vi "Enqueue Element.vi"(7 "timeout in ms (-1)":i32, 8 "error in":errorcluster, 9 "Element Placement":enum16{"To the Front", "To the Back"}(ring), 10 "Q Element":variant, 11 "QueueMessageTransport in":refnum<class "QueueMessageTransport.lvclass">) -> (0 "error out":errorcluster, 3 "QueueMessageTransport out":refnum<class "QueueMessageTransport.lvclass">)   [LabVIEW 2016, in "QueueMessageTransport.lvclass"]
doc: "This public method adds a queue element either <B>to the front</B> of the queue or <B>to the back</B>\n\n**Author: Stas Legedza"
uses:
  QueueMessageTransport.lvclass
  QueueMessageTransport.lvclass/QueueMessageTransport.ctl
panel:
  # "INPUTS"
  # "OUTPUTS"
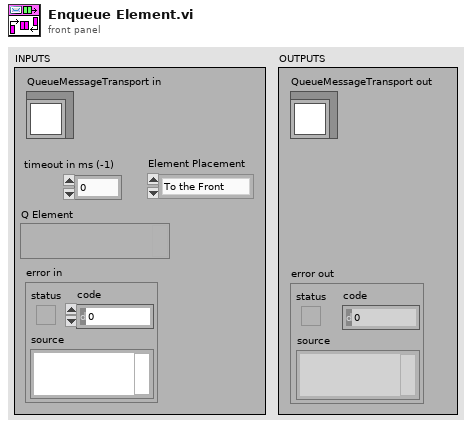
[diagram p1: front panel]
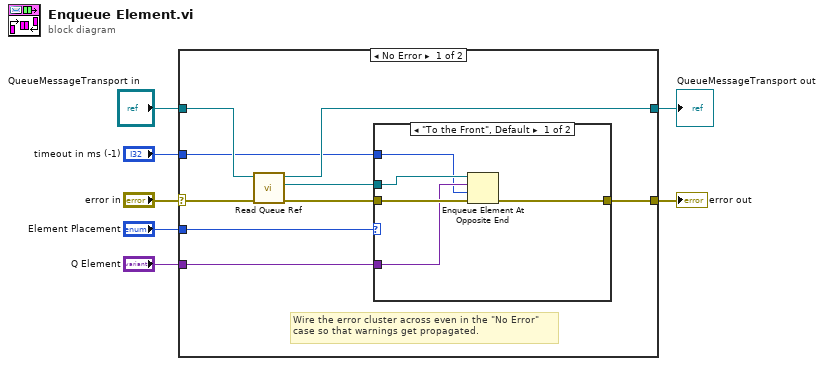
[diagram p0: block diagram]
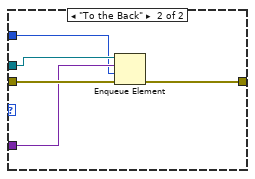
[diagram p2: hidden frame]
diagram:
  n1 = case shown="No Error" "error in" {
    selector: "error in" -> [w16 w28]
    tunnel: [w8 w28] -> w6
    tunnel: [w13 w27] -> w4
    tunnel: "QueueMessageTransport in" -> [w14 w27]
    tunnel: "Element Placement" -> [w15 _]
    tunnel: "Q Element" -> [w10 _]
    tunnel: "timeout in ms (-1)" -> [w9 _]
    frame No Error {
      # "Wire the error cluster across even in the \"No Error\"\ncase so that warnings get propagated."
      n2 = call "Read Queue Ref.vi"("error in"=w16, "QueueMessageTransport in"=w14) -> ("error out"=w11:errorcluster, "Queue Ref"=w12:refnum<queue>, "QueueMessageTransport out"=w13:refnum<class "QueueMessageTransport.lvclass">)  [unwired: 7 in]
      n3 = case shown="\"To the Front\", Default" w15 {
        tunnel: w12 -> [w20 w26]
        tunnel: w11 -> [w21 w25]
        tunnel: w10 -> [w19 w24]
        tunnel: w9 -> [w18 w23]
        tunnel: [w17 w22] -> w8
        frame "To the Front", Default {
          n4 = Enqueue Element At Opposite End(queue=w20, element=w19, timeout in ms (-1)=w18, error in (no error)=w21) -> (error out=w17:errorcluster)  [unwired: 2 out]
        }
        frame "To the Back" {
          n5 = Enqueue Element(queue=w26, element=w24, timeout in ms (-1)=w23, error in (no error)=w25) -> (error out=w22:errorcluster)  [unwired: 2 out]
        }
      }
    }
    frame Error {
    }
  }
  "error out" <- w6
  "QueueMessageTransport out" <- w4
